vi "Get Timeout (-1 infini).vi"(8 "error in (no error)":errorcluster caption="entrée d'erreur (pas d'erreur)", 11 "Server TCP_IP (Default) en entrée":refnum<class "Server TCP_IP (Default).lvclass">) -> (0 "error out":errorcluster caption="sortie d'erreur", 2 "Timeout (-1 infini)":i16, 3 "Server TCP_IP (Default) en sortie":refnum<class "Server TCP_IP (Default).lvclass">)   [LabVIEW 2020, in "Library Instrument & Equipement.lvlib" / "Library TCP IP.lvlib" / "Server TCP_IP (Default).lvclass"]
uses:
  Server TCP_IP (Default).lvclass
  Server TCP_IP (Default).lvclass/Server TCP_IP (Default).ctl
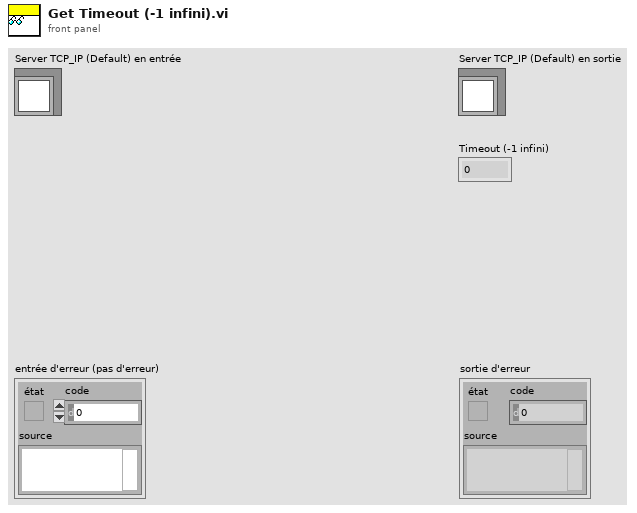
[diagram p1: front panel]
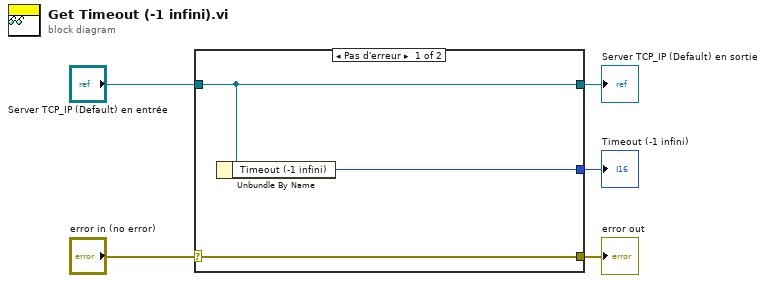
[diagram p0: block diagram]
diagram:
  n1 = case shown="Pas d'erreur" "error in (no error)" {
    selector: "error in (no error)" -> [w8 w9]
    tunnel: [w8 w9] -> w4
    tunnel: [w7 w10] -> w2
    tunnel: "Server TCP_IP (Default) en entrée" -> [w7 w10]
    tunnel: [w6 _] -> w1
    frame No Error {
      n2 = Unbundle By Name(w7) -> ("Timeout (-1 infini)"=w6:i16)
    }
    frame Error {
    }
  }
  "error out" <- w4
  "Server TCP_IP (Default) en sortie" <- w2
  "Timeout (-1 infini)" <- w1
